vi "DataSocket-Client.vi"() -> ()   [LabVIEW 2019]
doc: "Uses DataSocket to write array data. This example works for writing the data to the DataSocket Server (for live data). \n \nThe Writer, Server, and Reader can all be on the same computer or different computers. The Writer and Reader URLs should point to the computer where the DataSocket Server is."
panel:
  out "ProcState":enum16{"WaitCmd", "SelfTesting", "EndProc"}(ring)
  # "Overview: Demonstrates the use of the DataSocket functions to manage the remote client works\nRequirements: Windows\nInstructions:\n1. Run the DataSocket Server by navigating the Windows start menu to National Instruments > DataSocket > DataSocket Server.\n2. Run the DataSocket-Manager vi.\n3. Open and run DaraSocket-Client vi.\n4. Checkout the state change in indicator ProcState."
  # "DataSocket - Client"
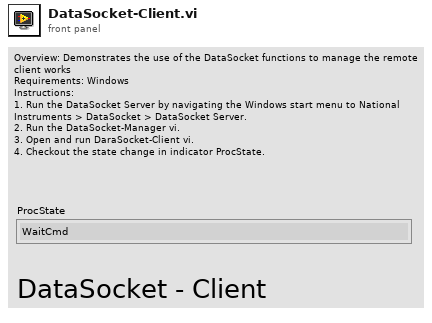
[diagram p1: front panel]
types:
  T1 = enum16{"Read", "Write", "ReadWrite", "BufferedRead", "BufferedReadWrite"}
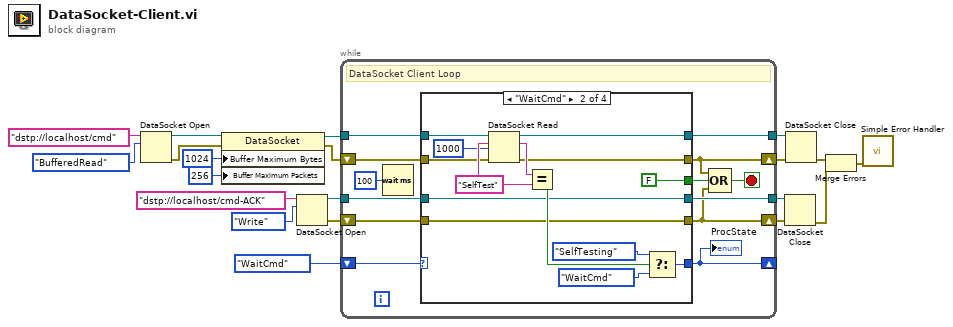
[diagram p0: block diagram]
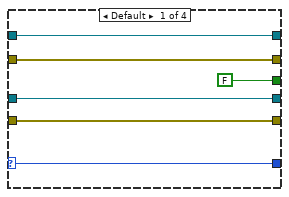
[diagram p2: hidden frame]
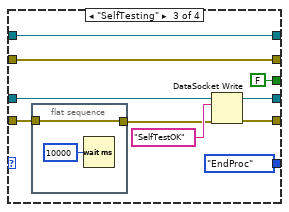
[diagram p3: hidden frame]
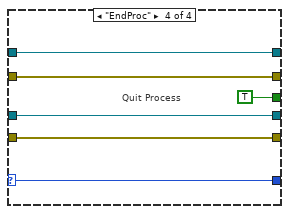
[diagram p4: hidden frame]
diagram:
  n1 = DataSocket Open(10:T1."BufferedRead" ("mode"), 11:"dstp://localhost/cmd" ("Write Location")) -> (0:w2:errorcluster, 3:w4:refnum<k13>)  [unwired: 2 in]
  n2 = property class="DataSocket"(reference=w4, error in=w2, "Buffer Maximum Bytes"=1024, "Buffer Maximum Packets"=256) -> (reference out=w3:refnum<k13>, error out=w1:errorcluster)
  n3 = DataSocket Open(10:T1."Write" ("mode"), 11:"dstp://localhost/cmd-ACK" ("Write Location")) -> (0:w11:errorcluster, 3:w13:refnum<k13>)  [unwired: 2 in]
  n4 = while {
    tunnel: w3 -> [w32]
    tunnel: [w30] -> w19
    tunnel: w13 -> [w28]
    tunnel: [w27] -> w12
    shift-right: [w21] -> _
    shift-left: enum16{"WaitCmd", "SelfTesting", "EndProc"}."WaitCmd" -> [w29]
    shift-right: [w24] -> w20
    shift-left: w1 -> [w33]
    shift-right: [w23] -> w10
    shift-left: w11 -> [w26]
    stop <- w25 stop-if-true
    # "DataSocket Client Loop"
    n5 = Wait (ms)(milliseconds to wait=u32 100) -> ()  [unwired: 1 out]
    n6 = case shown="\"WaitCmd\"" w29 {
      selector: w29 -> [w35 _ _ w66]
      tunnel: w33 -> [w38 w43 w57 w70]
      tunnel: w32 -> [w39 w45 w56 w71]
      tunnel: [w38 w42 w57 w70] -> w24
      tunnel: [w39 w44 w56 w71] -> w30
      tunnel: w28 -> [w37 w41 w60 w69]
      tunnel: [w37 w41 w58 w69] -> w27
      tunnel: [w35 w47 enum16{"WaitCmd", "SelfTesting", "EndProc"}."EndProc" w66] -> w21
      tunnel: w26 -> [w36 w40 w55 w68]
      tunnel: [w36 w40 w59 w68] -> w23
      tunnel: [FALSE FALSE FALSE TRUE] -> w22
      frame Default {
      }
      frame "WaitCmd" {
        w52 = "SelfTest"
        n7 = DataSocket Read(8:w43, 9:1000 ("ms timeout (10000)"), 10:w52, 11:w45) -> (0:w42:errorcluster, 2:w53:string, 3:w44:refnum<k13>)  [unwired: 1 in, 4 out]
        n8 = Equal?(x=w53, y=w52) -> (x = y?=w50:bool)
        n9 = Select(t=enum16{"WaitCmd", "SelfTesting", "EndProc"}."SelfTesting", s=w50, f=enum16{"WaitCmd", "SelfTesting", "EndProc"}."WaitCmd") -> (s? t:f=w47:enum16{"WaitCmd", "SelfTesting", "EndProc"})
      }
      frame "SelfTesting" {
        n10 = flat-sequence {
          tunnel: [w65] -> w54
          tunnel: w55 -> [w65]
          frame #0 {
            n11 = Wait (ms)(milliseconds to wait=u32 10000) -> ()  [unwired: 1 out]
          }
        }
        n12 = DataSocket Write(8:w54, 10:"SelfTestOK", 11:w60) -> (0:w59:errorcluster, 3:w58:refnum<k13>)  [unwired: 2 out]
      }
      frame "EndProc" {
        # "Quit Process"
      }
    }
    "ProcState" <- w21
    n13 = Compound Arithmetic op=OR(w24, w22, w23) -> (w25:bool)
  }
  n14 = DataSocket Close(8:w10, 11:w12) -> (0:w7:errorcluster)  [unwired: 1 in, 1 out]
  n15 = DataSocket Close(8:w20, 11:w19) -> (0:w8:errorcluster)  [unwired: 1 in, 1 out]
  n16 = Merge Errors(w8, w7) -> (w9:errorcluster)
  n17 = call <vilib>:"Simple Error Handler.vi"("error in (no error)"=w9) -> ()  [unwired: 4 in, 5 out]
